vi "test json path.vi"(8 "error in (no error)":errorcluster) -> (0 "error out":errorcluster)   [LabVIEW 2019, in "labview_json_tests.lvlib"]
uses:
  labview_json_tests.lvlib
  lib/Element Type.ctl
  lib/labview_json.lvlib
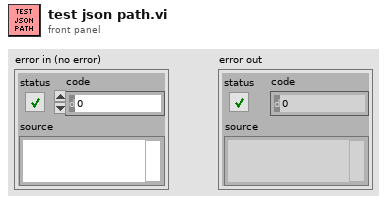
[diagram p1: front panel]
types:
  T1 = typedef "labview_json.lvlib/Element Type.ctl" = enum8{"NULL", "OBJECT", "ARRAY", "BOOL", "INT", "UINT", "FLOAT", "STRING"}
  T2 = typedef "labview_json.lvlib/Element.ctl" = cluster{"Key":string, "Type":T1, "Value":variant}
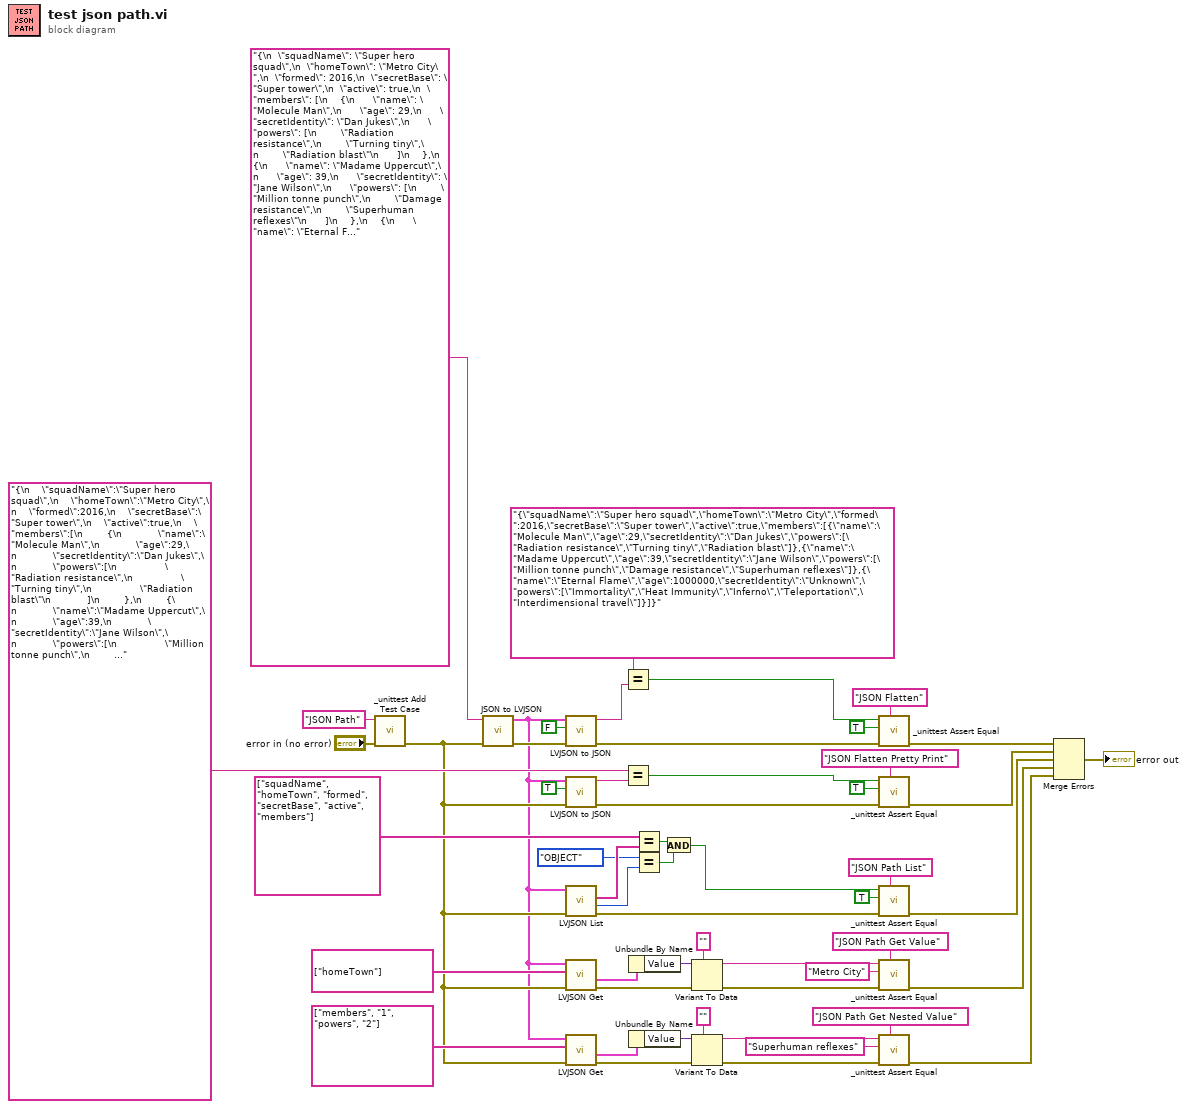
[diagram p0: block diagram]
diagram:
  n1 = call "_unittest Add Test Case.vi"("error in (no error)"="error in (no error)", "Test Case"="JSON Path") -> ("error out"=w3:errorcluster)  [unwired: 9 in]
  n2 = call "JSON to LVJSON.vi"("error in (no error)"=w3, "JSON"="{\n  \"squadName\": \"Super hero squad\",\n  \"homeTown\": \"Metro City\",\n  \"formed\": 2016,\n  \"secretBase\": \"Super tower\",\n  \"active\": true,\n  \"members\": [\n    {\n      \"name\": \"Molecule Man\",\n      \"age\": 29,\n      \"secretIdentity\": \"Dan Jukes\",\n      \"powers\": [\n        \"Radiation resistance\",\n        \"Turning tiny\",\n        \"Radiation blast\"\n      ]\n    },\n    {\n      \"name\": \"Madame Uppercut\",\n      \"age\": 39,\n      \"secretIdentity\": \"Jane Wilson\",\n      \"powers\": [\n        \"Million tonne punch\",\n        \"Damage resistance\",\n        \"Superhuman reflexes\"\n      ]\n    },\n    {\n      \"name\": \"Eternal Flame\",\n      \"age\": 1000000,\n      \"secretIdentity\": \"Unknown\",\n      \"powers\": [\n        \"Immortality\",\n        \"Heat Immunity\",\n        \"Inferno\",\n        \"Teleportation\",\n        \"Interdimensional travel\"\n      ]\n    }\n  ]\n}") -> ("error out"=w47:errorcluster, "Root Element"=w2:T2)  [unwired: 8 in]
  n3 = call "LVJSON to JSON.vi"("error in (no error)"=w47, "Pretty Print? (F)"=FALSE, "Root"=w2) -> ("error out"=w46:errorcluster, "JSON"=w44:string)  [unwired: 6 in, 1 out]
  n4 = call "LVJSON to JSON.vi"("error in (no error)"=w3, "Pretty Print? (F)"=TRUE, "Root"=w2) -> ("error out"=w35:errorcluster, "JSON"=w37:string)  [unwired: 6 in, 1 out]
  n5 = call "LVJSON List.vi"("error in (no error)"=w3, "Root in"=w2) -> ("error out"=w30:errorcluster, "Type"=w28:T1, "Keys/Indexes"=w29:string[])  [unwired: 6 in, 1 out]
  n6 = call "LVJSON Get.vi"("error in (no error)"=w3, "JSON Path"=string[] ["homeTown"], "Root in"=w2) -> ("error out"=w20:errorcluster, "Value"=w18:T2)  [unwired: 5 in, 2 out]
  n7 = call "LVJSON Get.vi"("error in (no error)"=w3, "JSON Path"=string[] ["members", "1", "powers", "2"], "Root in"=w2) -> ("error out"=w6:errorcluster, "Value"=w7:T2)  [unwired: 5 in, 2 out]
  n8 = Equal?(x="{\"squadName\":\"Super hero squad\",\"homeTown\":\"Metro City\",\"formed\":2016,\"secretBase\":\"Super tower\",\"active\":true,\"members\":[{\"name\":\"Molecule Man\",\"age\":29,\"secretIdentity\":\"Dan Jukes\",\"powers\":[\"Radiation resistance\",\"Turning tiny\",\"Radiation blast\"]},{\"name\":\"Madame Uppercut\",\"age\":39,\"secretIdentity\":\"Jane Wilson\",\"powers\":[\"Million tonne punch\",\"Damage resistance\",\"Superhuman reflexes\"]},{\"name\":\"Eternal Flame\",\"age\":1000000,\"secretIdentity\":\"Unknown\",\"powers\":[\"Immortality\",\"Heat Immunity\",\"Inferno\",\"Teleportation\",\"Interdimensional travel\"]}]}" ("JSON"), y=w44) -> (x = y?=w41:bool)
  n9 = Equal?(x="{\n    \"squadName\":\"Super hero squad\",\n    \"homeTown\":\"Metro City\",\n    \"formed\":2016,\n    \"secretBase\":\"Super tower\",\n    \"active\":true,\n    \"members\":[\n        {\n            \"name\":\"Molecule Man\",\n            \"age\":29,\n            \"secretIdentity\":\"Dan Jukes\",\n            \"powers\":[\n                \"Radiation resistance\",\n                \"Turning tiny\",\n                \"Radiation blast\"\n            ]\n        },\n        {\n            \"name\":\"Madame Uppercut\",\n            \"age\":39,\n            \"secretIdentity\":\"Jane Wilson\",\n            \"powers\":[\n                \"Million tonne punch\",\n                \"Damage resistance\",\n                \"Superhuman reflexes\"\n            ]\n        },\n        {\n            \"name\":\"Eternal Flame\",\n            \"age\":1000000,\n            \"secretIdentity\":\"Unknown\",\n            \"powers\":[\n                \"Immortality\",\n                \"Heat Immunity\",\n                \"Inferno\",\n                \"Teleportation\",\n                \"Interdimensional travel\"\n            ]\n        }\n    ]\n}" ("JSON"), y=w37) -> (x = y?=w39:bool)
  n10 = Unbundle By Name(w18) -> ("Value"=w16:variant)
  n11 = Unbundle By Name(w7) -> ("Value"=w9:variant)
  n12 = Equal?(x=string[] ["squadName", "homeTown", "formed", "secretBase", "active", "members"], y=w29) -> (x = y?=w25:bool)
  n13 = Equal?(x=Element_Type."OBJECT", y=w28) -> (x = y?=w24:bool)
  n14 = And(x=w25, y=w24) -> (x .and. y?=w23:bool)
  n15 = Variant To Data(error in=w20, type="", Variant=w16) -> (data=w14:string, error out=w17:errorcluster)
  n16 = Variant To Data(error in=w6, type="", Variant=w9) -> (data=w11:string, error out=w8:errorcluster)
  n17 = call "_unittest Assert Equal.vi"("Message"="JSON Flatten", "error in (no error)"=w46, "Expected Value"=TRUE, "Actual Value"=w41) -> ("error out"=w52:errorcluster)  [unwired: 7 in]
  n18 = call "_unittest Assert Equal.vi"("Message"="JSON Flatten Pretty Print", "error in (no error)"=w35, "Expected Value"=TRUE, "Actual Value"=w39) -> ("error out"=w33:errorcluster)  [unwired: 7 in]
  n19 = call "_unittest Assert Equal.vi"("Message"="JSON Path List", "error in (no error)"=w30, "Expected Value"=TRUE, "Actual Value"=w23) -> ("error out"=w32:errorcluster)  [unwired: 7 in]
  n20 = call "_unittest Assert Equal.vi"("Message"="JSON Path Get Value", "error in (no error)"=w17, "Expected Value"="Metro City", "Actual Value"=w14) -> ("error out"=w19:errorcluster)  [unwired: 7 in]
  n21 = call "_unittest Assert Equal.vi"("Message"="JSON Path Get Nested Value", "error in (no error)"=w8, "Expected Value"="Superhuman reflexes", "Actual Value"=w11) -> ("error out"=w1:errorcluster)  [unwired: 7 in]
  n22 = Merge Errors(w52, w33, w32, w19, w1) -> (→"error out":errorcluster)
